vi "Is_PackedItem.vi"(8 "error in (no error)":errorcluster, 11 "AB_Source_PackedItem in":refnum<class "AB_Source_PackedItem.lvclass">) -> (0 "error out":errorcluster, 2 "packed item":bool, 3 "AB_Source_PackedItem out":refnum<class "AB_Source_PackedItem.lvclass">)   [LabVIEW 2020, in "AB_Source_PackedItem.lvclass"]
uses:
  <vilib>/AppBuilder/AB_Classes/Source/PackedItem/AB_Source_PackedItem.lvclass
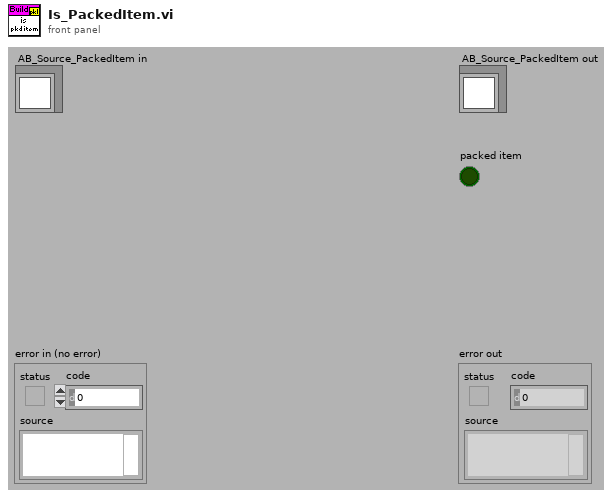
[diagram p1: front panel]
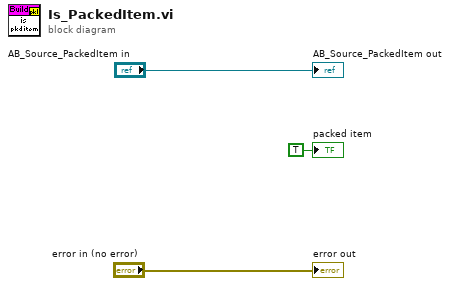
[diagram p0: block diagram]
diagram:
  "error out" <- "error in (no error)"
  "AB_Source_PackedItem out" <- "AB_Source_PackedItem in"
  "packed item" <- TRUE ("packed item")
